vi "In Range.vi"(5 "Range":dbl, 7 "Setpoint":dbl, 11 "Value":dbl) -> (3 "in range?":bool)   [LabVIEW 2019]
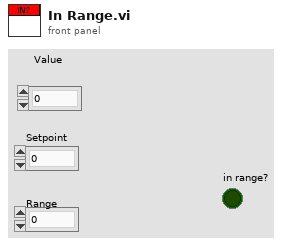
[diagram p1: front panel]
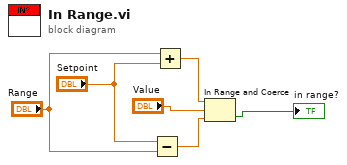
[diagram p0: block diagram]
diagram:
  n1 = Subtract(x="Setpoint", y="Range") -> (x-y=w5:dbl)
  n2 = Add(x="Range", y="Setpoint") -> (x+y=w6:dbl)
  n3 = In Range and Coerce(upper limit=w6, x="Value", lower limit=w5) -> (In Range?=→"in range?":bool)  [unwired: 1 out]
